vi "setEndTone.vi"(8 "error in (no error)":errorcluster, 10 "endTone":refnum<class "SingleTone.lvclass">, 11 "RampTone.lvclass in":refnum<class "RampTone.lvclass">) -> (0 "error out":errorcluster, 3 "RampTone.lvclass out":refnum<class "RampTone.lvclass">)   [LabVIEW 2011, in "Tools.lvlib" / "Scripting.lvlib" / "RampTone.lvclass"]
uses:
  RampTone.lvclass
  SingleTone/SingleTone.lvclass
  RampTone.lvclass/RampTone.ctl
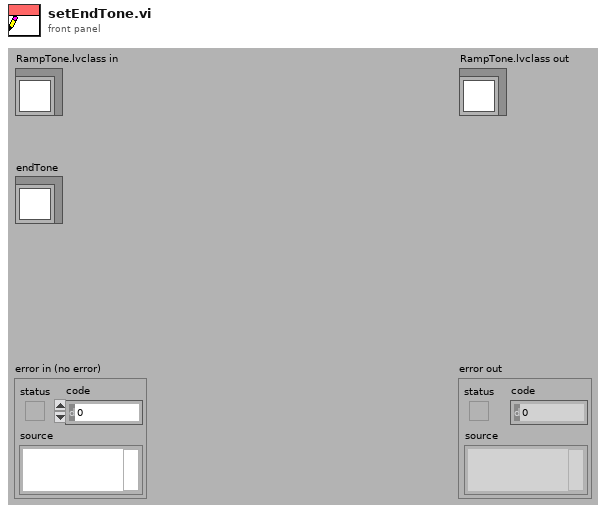
[diagram p1: front panel]
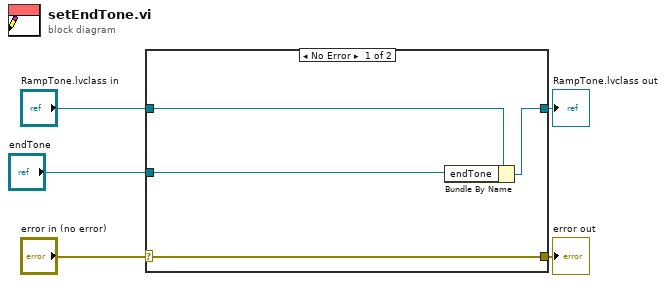
[diagram p0: block diagram]
diagram:
  n1 = case shown="No Error" "error in (no error)" {
    selector: "error in (no error)" -> [w9 w10]
    tunnel: [w9 w10] -> w4
    tunnel: [w7 w11] -> w2
    tunnel: "RampTone.lvclass in" -> [w8 w11]
    tunnel: "endTone" -> [w6 _]
    frame No Error {
      n2 = Bundle By Name(cluster=w8, "endTone"=w6) -> (w7:refnum<class "RampTone.lvclass">)
    }
    frame Error {
    }
  }
  "error out" <- w4
  "RampTone.lvclass out" <- w2
